vi "Generate Channel Mappings.vi"(7 "Starting Buffer Offset (0)":u64, 8 "error in (no error)":errorcluster, 9 "Plugin Data Offset":T3 format="%.0x", 10 "Channels":T2[](array[typedef]), 11 "Simulated VeriStand Engine in":refnum<class "Simulated VeriStand Engine.lvclass">) -> (0 "error out":errorcluster, 1 "Base Pointer":u64 format="%016x", 2 "mappings":T1[](array[typedef]), 3 "Simulated VeriStand Engine out":refnum<class "Simulated VeriStand Engine.lvclass">)   [LabVIEW 2016, in "Simulated VeriStand Engine.lvclass"]
uses:
  Simulated VeriStand Engine.lvclass
  <vilib>/NI Veristand/Custom Device API/Data Reference.ctl
  <vilib>/NI Veristand/VeriStand Data/Typedefs/Typedefs.Data Types.ctl
  <vilib>/NI Veristand/VeriStand Data/Byte Buffer/Byte Buffer.Mapping.ctl
  <vilib>/NI Veristand/VeriStand Data/Data Channels/Channels.Inline.Reference Error Handler.vi
  <vilib>/NI Veristand/Custom Device API/Global Data Refs.vi
  <vilib>/NI Veristand/VeriStand Data/VeriStand Data.lvlib
  <vilib>/NI Veristand/VeriStand Data/Byte Buffer/Byte Buffer.lvclass
  <vilib>/NI VeriStand/Custom Device API/Custom Device API.lvlib
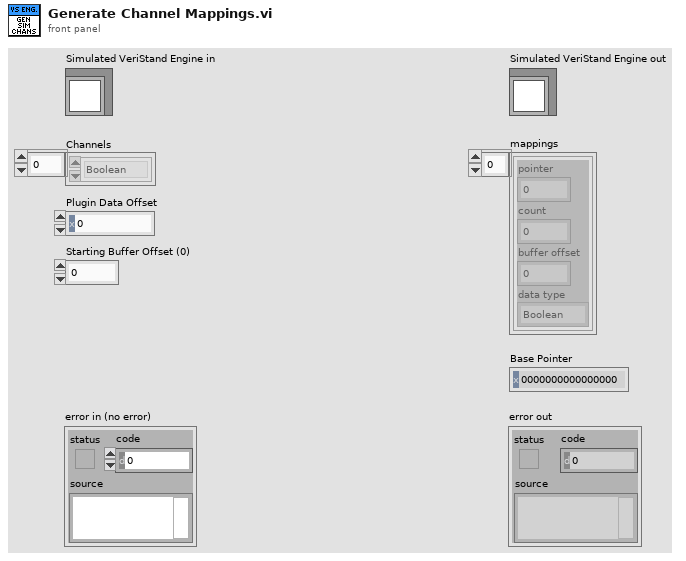
[diagram p1: front panel]
types:
  T1 = typedef "VeriStand Data.lvlib/Byte Buffer.lvclass/Byte Buffer.Mapping.ctl" = cluster{"pointer":u64, "count":i64, "buffer offset":u64, "data type":T2}
  T2 = typedef "VeriStand Data.lvlib/Typedefs.Data Types.ctl" = enum16{"Boolean", "Single", "Double", "I8", "I16", "I32", "I64", "U8", "U16", "U32", "U64"}
  T3 = typedef "Custom Device API.lvlib/Data Reference.ctl" = i32
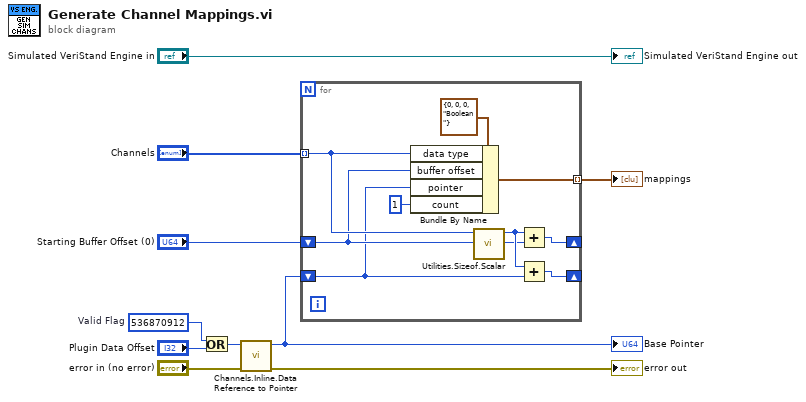
[diagram p0: block diagram]
diagram:
  w9 = T3 536870912  # Valid Flag
  n1 = Or(x=w9, y="Plugin Data Offset") -> (x .or. y?=w8:T3)
  n2 = call <vilib>:"Channels.Inline.Data Reference to Pointer.vi"("error in (no error)"="error in (no error)", "Data Reference in"=w8) -> ("error out"=→"error out":errorcluster, "Channel Pointer"=w6:u64)  [unwired: 8 in]
  "Base Pointer" <- w6
  n3 = for {
    shift-right: [w18] -> _
    shift-left: "Starting Buffer Offset (0)" -> [w14]
    shift-right: [w16] -> _
    shift-left: w6 -> [w13]
    tunnel: "Channels" -> [w15] mode=indexing
    tunnel: [w11] -> w2 mode=indexing
    n4 = Bundle By Name(cluster=T1 {"pointer"=0, "count"=0, "buffer offset"=0, "data type"=enum."Boolean"} ("mapping"), "data type"=w15, "buffer offset"=w14, "pointer"=w13, "count"=i64 1) -> (w11:T1)
    n5 = call <vilib>:"Utilities.Sizeof.Scalar.vi"("data type"=w15) -> ("size in bytes"=w17:u64)  [unwired: 9 in, 1 out]
    n6 = Add(x=w17, y=w14) -> (x+y=w18:u64)
    n7 = Add(x=w17, y=w13) -> (x+y=w16:u64)
  }
  "mappings" <- w2
  "Simulated VeriStand Engine out" <- "Simulated VeriStand Engine in"
